vi "Set SR List Position and Size.vi"(4 "FP.width":i16, 6 "FP.height":i16, 8 "error in":errorcluster, 10 "label array in":string[](array[string]), 11 "controls[] in":refnum<vi>[](array[refnum])) -> (0 "error out":errorcluster, 1 "SR List.height":u32, 2 "label array out":string[](array[string]), 3 "controls[] out":refnum<vi>[](array[refnum]))   [LabVIEW 2018]
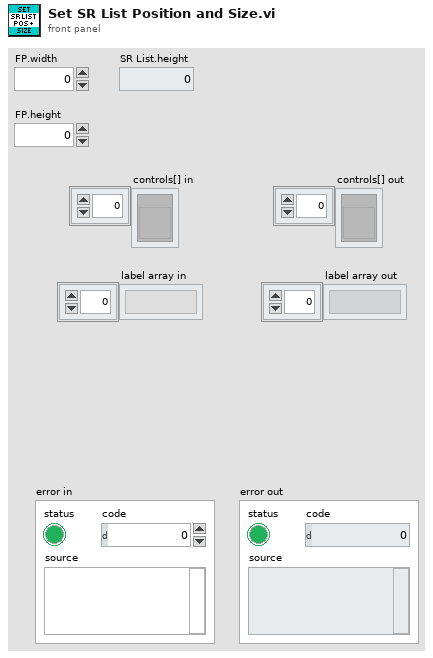
[diagram p1: front panel]
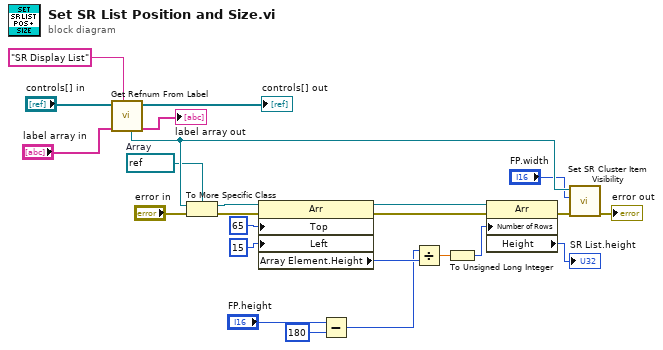
[diagram p0: block diagram]
diagram:
  w12 = refnum<vi> refnum  # Array
  n1 = call "Get Refnum From Label.vi"("label"="SR Display List" ("element"), "label array in"="label array in", "controls[] in"="controls[] in") -> ("label array out"=→"label array out":string[], "controls[] out"=→"controls[] out":refnum<vi>[], "refnum out"=w22:refnum<vi>)  [unwired: 6 in]
  n2 = To More Specific Class(target class=w12, reference=w22, error in="error in") -> (specific class reference=w19:refnum<vi>, error out=w13:errorcluster)
  n3 = property class="Arr"(reference=w19, error in=w13, "Top"=65 ("Position:Top"), "Left"=15 ("Position:Left")) -> (reference out=w15:refnum<vi>, error out=w24:errorcluster, "Array Element.Height"=w16:u32)
  n4 = Subtract(x="FP.height", y=i16 180) -> (x-y=w2:i16)
  n5 = Divide(x=w2, y=w16) -> (x/y=w20:dbl)
  n6 = To Unsigned Long Integer(number=w20) -> (unsigned 32bit integer=w21:u32)
  n7 = property class="Arr"(reference=w15, error in=w24, "Number of Rows"=w21) -> (error out=w23:errorcluster, "Height"=→"SR List.height":u32)  [unwired: 1 out]
  n8 = call "Set SR Cluster Item Visibility.vi"("error in"=w23, "Screen Width"="FP.width", "SR List ref in"=w22) -> ("error out"=→"error out":errorcluster)  [unwired: 8 in]
